vi "Flatten.vi"(8 "error in (no error)":errorcluster, 11 "Function Gen Scan in":refnum<class "Function Gen Scan.lvclass">) -> (0 "error out":errorcluster, 3 "Function Gen Scan out":refnum<class "Function Gen Scan.lvclass">)   [LabVIEW 2017, in "Function Gen Scan.lvclass"]
uses:
  Function Gen Scan.lvclass
  Function Gen Scan.lvclass/Function Gen Scan.ctl
  Global/File Locations.vi
  Scanner/Scanner.lvclass
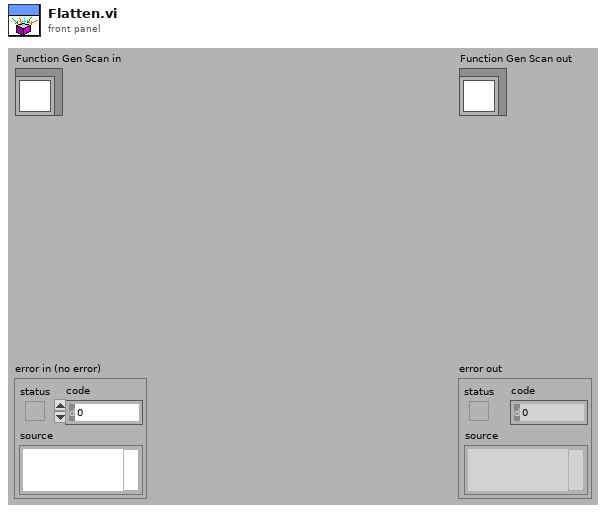
[diagram p1: front panel]
types:
  T1 = typedef "Channel.ctl" = u16
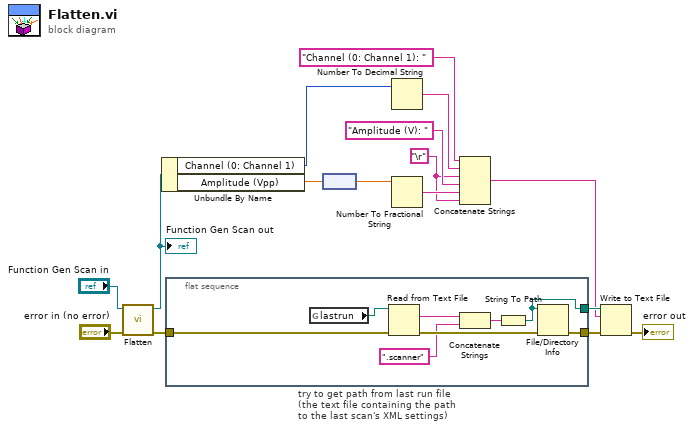
[diagram p0: block diagram]
diagram:
  w1 = "\r"
  n1 = call-parent "Flatten.vi"("error in (no error)"="error in (no error)", "Scanner in"="Function Gen Scan in") -> ("error out"=w14:errorcluster, "Scanner out"=w11:refnum<class "Function Gen Scan.lvclass">)  [unwired: 8 in]
  "Function Gen Scan out" <- w11
  n2 = Unbundle By Name(w11) -> ("Channel (0: Channel 1)"=w10:T1, "Amplitude (Vpp)"=w9:dbl[unit])
  n3 = flat-sequence "try to get path from last run file\n(the text file containing the path\nto the last scan's XML settings)" {
    tunnel: [w24] -> w6
    tunnel: [w21] -> w12
    tunnel: w14 -> [w17]
    frame #0 {
      n4 = global read "File Locations.vi" "lastrun"() -> (w23:path)
      n5 = Read from Text File(file (use dialog)=w23, error in=w17) -> (text=w20:string, error out=w22:errorcluster)  [unwired: 4 out]
      n6 = Concatenate Strings(w20, ".scanner") -> (w18:string)
      n7 = String To Path(string=w18) -> (path=w24:path)
      n8 = File/Directory Info(path=w24, error in=w22) -> (error out=w21:errorcluster)  [unwired: 6 out]
    }
  }
  n9 = node(w9) -> (w8:dbl)
  n10 = Number To Decimal String(number=w10) -> (decimal integer string=w4:string)  [unwired: 1 in]
  n11 = Number To Fractional String(number=w8) -> (F-format string=w3:string)  [unwired: 3 in]
  n12 = Concatenate Strings("Channel (0: Channel 1): ", w4, w1, "Amplitude (V): ", w3, w1) -> (w5:string)
  n13 = Write to Text File(file (use dialog)=w6, text=w5, error in=w12) -> (error out=→"error out":errorcluster)  [unwired: 1 in, 2 out]
